vi "ProcessCommand.vi"(5 "Ctl Refnum":refnum<vi>, 7 "Command":variant, 8 "error in (no error)":errorcluster, 9 "Data":T1=variant(string "Default"), 10 "Queue with Cluster Reference":T2, 11 "UserInput Command in":refnum<class "UserInput Command.lvclass">) -> (0 "error out":errorcluster, 2 "Queue (dup)":T2, 3 "UserInput Command out":refnum<class "UserInput Command.lvclass">)   [LabVIEW 2010, in "UserInput Command.lvclass"]
doc: "This VI serves as the dynamic dispatch VI for UserInput Commands.\n\nInputs:\nUserInput Command in - object used for commands from the user interface\n\nCommand - variant data type\n - not valid for valid control reference inputs\n - valid as string for Not A Ref on control reference input\n\nData - variant type that whose value can be used to override the control current value being placed in the queue with the command string\n\nQueue with Cluster Reference - reference to the EVM queue for inserting commands\n\nCtl Refnum - reference to the control that triggered the event; Not A Ref constant allows user defined string constants to be wired to Data input\nerror in - error input cluster\n\nOutputs:\nUserInput Command out - input object passed through\nQueue (dup) - input queue reference passed through\nerror out - error output cluster"
uses:
  UserInput Command.lvclass
  <userlib>/Common/Queue with Cluster/TYP_Queue with Cluster Reference.ctl
  Controls/TYP_VariantDefault.ctl
  UserInput Command.lvclass/UserInput Command.ctl
  <userlib>/Common/Queue with Cluster/Enqueue - ClusterBoth.vi
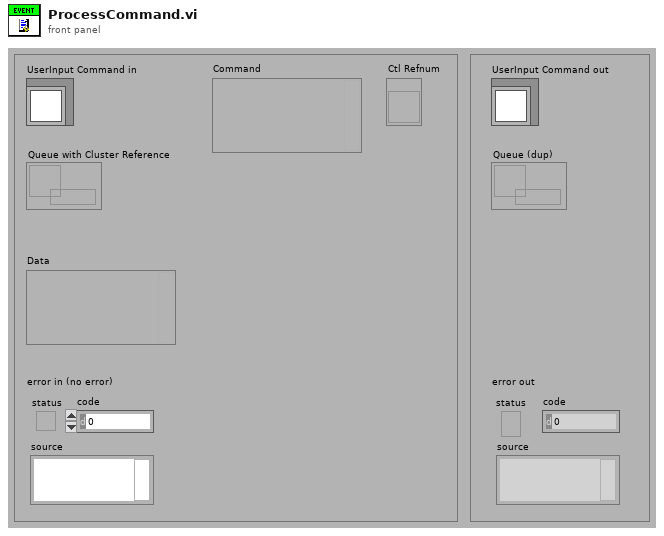
[diagram p1: front panel]
types:
  T1 = typedef "TYP_VariantDefault.ctl" = variant
  T2 = typedef "TYP_Queue with Cluster Reference.ctl" = refnum<queue>
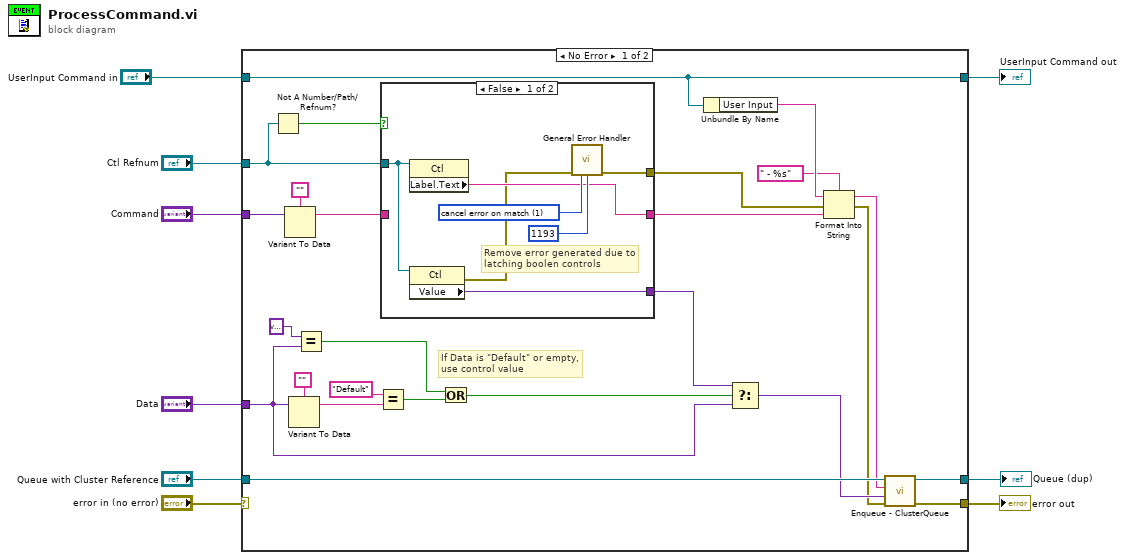
[diagram p0: block diagram]
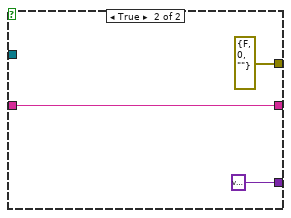
[diagram p2: hidden frame]
diagram:
  n1 = case shown="No Error" "error in (no error)" {
    selector: "error in (no error)" -> [_ w47]
    tunnel: [w34 w47] -> w8
    tunnel: [w31 w46] -> w6
    tunnel: "UserInput Command in" -> [w31 w46]
    tunnel: "Queue with Cluster Reference" -> [w33 w45]
    tunnel: [w32 w45] -> w4
    tunnel: "Ctl Refnum" -> [w17 _]
    tunnel: "Command" -> [w30 _]
    tunnel: "Data" -> [w15 _]
    frame No Error {
      # "If Data is \"Default\" or empty,\nuse control value"
      n2 = Not A Number/Path/Refnum?(number/path/refnum=w17) -> (NaN/Path/Refnum?=w10:bool)
      n3 = Variant To Data(Variant=w30, type="") -> (data=w28:string)  [unwired: 1 in, 1 out]
      n4 = Variant To Data(Variant=w15, type="") -> (data=w21:string)  [unwired: 1 in, 1 out]
      n5 = Equal?(x=variant ("Value"), y=w15) -> (x = y?=w14:bool)
      n6 = Equal?(x="Default", y=w21) -> (x = y?=w13:bool)
      n7 = case shown="False" w10 {
        tunnel: w28 -> [_ w44]
        tunnel: [w37 w44] -> w25
        tunnel: [w40 variant ("Value")] -> w18
        tunnel: w17 -> [w36 _]
        tunnel: [w38 errorcluster {"status"=FALSE, "code"=0, "source"=""} ("error out")] -> w11
        frame False {
          w41 = 1 items=["no exception", "cancel error on match", "set error on match"] ("[exception action] (none:0)")
          # "Remove error generated due to\nlatching boolen controls"
          n8 = property class="Ctl"(reference=w36) -> ("Label.Text"=w37:string)  [unwired: 1 in, 2 out]
          n9 = property class="Ctl"(reference=w36) -> (error out=w35:errorcluster, "Value"=w40:variant)  [unwired: 1 in, 1 out]
          n10 = call <vilib>:"General Error Handler.vi"("error in (no error)"=w35, "[exception action] (none:0)"=w41, "[exception code]"=1193) -> ("error out"=w38:errorcluster)  [unwired: 8 in, 4 out]
        }
        frame True {
        }
      }
      n11 = Or(x=w14, y=w13) -> (x .or. y?=w12:bool)
      n12 = Unbundle By Name(w31) -> ("User Input"=w27:string)
      n13 = Select(t=w18, s=w12, f=w15) -> (s? t:f=w22:T1)
      n14 = Format Into String(format string=" - %s", initial string=w27, error in=w11, w25) -> (resulting string=w24:string, error out=w19:errorcluster)
      n15 = call-poly <userlib>:"Enqueue - ClusterQueue.vi"("error in (no error)"=w19, "Data"=w22, "Command"=w24, "Queue with Cluster Reference"=w33) -> ("error out"=w34:errorcluster, "Queue Out (dup)"=w32:T2)  [unwired: 6 in]
    }
    frame Error {
    }
  }
  "error out" <- w8
  "UserInput Command out" <- w6
  "Queue (dup)" <- w4
